vi "Interrogate_register.vi"(6 "Address override":i32, 8 "error in (no error)":errorcluster, 9 "UUT Index":i32, 10 "Register mutli-protocol location":T2={"General Parameter name"="", "MODBUS Register"=0, "Profibus"={"Friendly name"="", "PA"={"Slot"=0, "Index"=0}, "DP"={"Slot"=0, "Index"=0}, "Tag"=""}, "Fieldbus"={"Parameter name"="", "Fieldbus Block"="", "Fieldbus Tag"=""}, "data type"=enum."float", "DeviceNET"={"ClassId"=102, "InstanceId"=1, "AttributeId"=12}, "Cluster"={"address"=0, "Mode"=0}, "Length"=0} {"Cluster"."Mode" items=["None", "MODBUS", "HART", "Profibus DP", "Profibus PA", "Fieldbus", "DeviceNET"]}, 11 "HART in":refnum<class "HART.lvclass">) -> (0 "error out":errorcluster, 1 "Parameter name":string, 2 "output":sgl, 3 "HART out":refnum<class "HART.lvclass">, 4 "output cluster":T1)   [LabVIEW 2016, in "HART.lvclass"]
uses:
  HART.lvclass
  Typedef/comm_variable_definition.ctl
  Typedef/Comm_mode_and_address_type.ctl
  Typedef/Comm_mode_type_combo.ctl
  HART.lvclass/HART.ctl
  Protocol Class/Protocol.lvclass
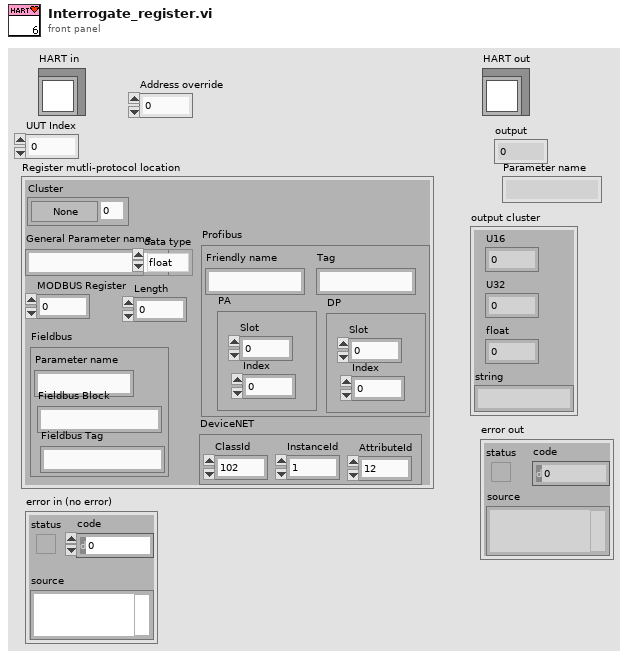
[diagram p1: front panel]
types:
  T1 = cluster{"U16":u16, "U32":u32, "float":sgl, "string":string}
  T2 = typedef "comm_variable_definition.ctl" = cluster{"General Parameter name":string, "MODBUS Register":i32, "Profibus":cluster{"Friendly name":string, "PA":cluster{"Slot":i32, "Index":i32}, "DP":cluster{"Slot":i32, "Index":i32}, "Tag":string}, "Fieldbus":cluster{"Parameter name":string, "Fieldbus Block":string, "Fieldbus Tag":string}, "data type":enum16{"float", "UINT", "UINT32", "STRING"}, "DeviceNET":cluster{"ClassId":u16, "InstanceId":u16, "AttributeId":u8}, "Cluster":T3, "Length":i32}
  T3 = typedef "Comm_mode_and_address_type.ctl" = cluster{"address":i32, "Mode":T4}
  T4 = typedef "Comm_mode_type_combo.ctl" = u16
  T5 = enum16{"None", "Coil", "Uint16", "Uint32", "Float"}
  T6 = enum16{"0-1-2-3", "2-3-0-1", "1-0-3-2", "3-2-1-0"}
  T7 = cluster{"Long address":u8[], "Short address":i32, "Switch index":i32}[]
  T8 = cluster{"Long address":u8[], "Short address":i32, "Switch index":i32}
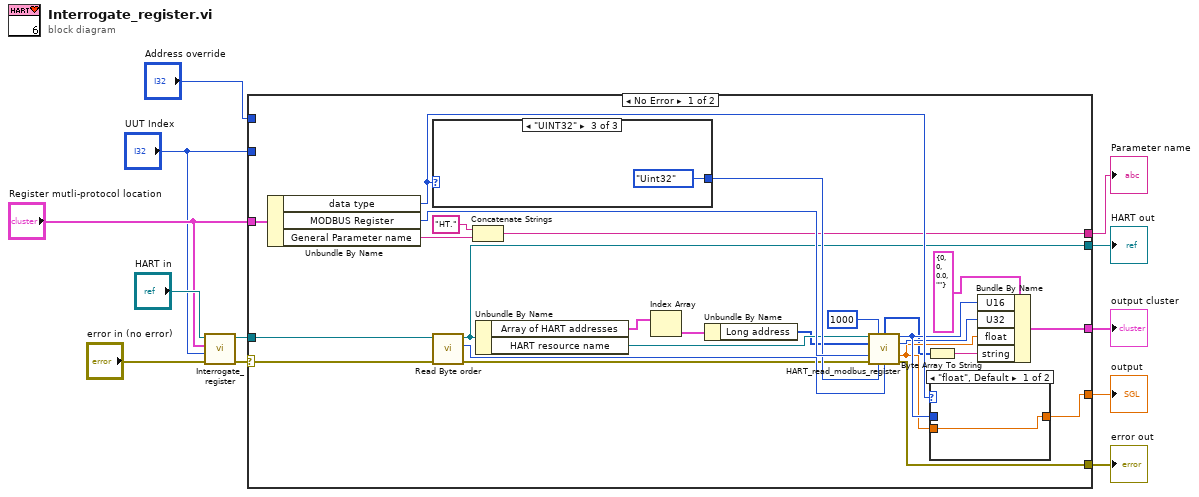
[diagram p0: block diagram]
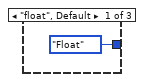
[diagram p3: hidden frame]
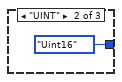
[diagram p4: hidden frame]
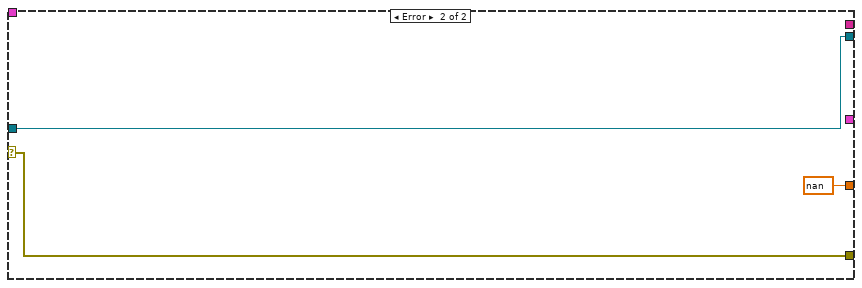
[diagram p5: hidden frame]
diagram:
  n1 = call-parent "Interrogate_register.vi"("error in (no error)"="error in (no error)", "UUT Index"="UUT Index", "Register mutli-protocol location"="Register mutli-protocol location", "Protocol in"="HART in") -> ("error out"=w10:errorcluster, "Protocol out"=w9:refnum<class "HART.lvclass">)  [unwired: 3 in, 3 out]
  n2 = case shown="No Error" w10 {
    selector: w10 -> [w14 w46]
    tunnel: "Register mutli-protocol location" -> [w38 _]
    tunnel: [w37 sgl nan ("type single")] -> w4
    tunnel: [w34 w46] -> w5
    tunnel: "UUT Index" -> [_ _]
    tunnel: w9 -> [w17 w44]
    tunnel: [w16 w44] -> w6
    tunnel: [w25 _] -> w3
    tunnel: "Address override" -> [_ _]
    tunnel: [w18 _] -> w1
    frame No Error {
      n3 = Unbundle By Name(w38) -> ("data type"=w36:enum16{"float", "UINT", "UINT32", "STRING"}, "MODBUS Register"=w35:i32, "General Parameter name"=w26:string)
      n4 = case shown="\"UINT32\"" w36 {
        tunnel: [T5."Float" ("data type") T5."Uint16" ("data type") T5."Uint32" ("data type")] -> w33
        frame "float", Default {
        }
        frame "UINT" {
        }
        frame "UINT32" {
        }
      }
      n5 = call-dynamic "Read Byte order.vi"("error in (no error)"=w14, "Protocol in"=w17) -> ("error out"=w13:errorcluster, "Byte order"=w15:T6, "Protocol out"=w16:refnum<class "HART.lvclass">)  [unwired: 7 in]
      n6 = Concatenate Strings("HT." ("Protocol name"), w26) -> (w25:string)
      n7 = Unbundle By Name(w16) -> ("Array of HART addresses"=w31:T7, "HART resource name"=w32:refnum<visa-resource-name>)
      n8 = Index Array(array=w31) -> (element=w30:T8)  [unwired: 1 in]
      n9 = Unbundle By Name(w30) -> ("Long address"=w29:u8[])
      n10 = call "HART_read_modbus_register.vi"("port number"=w32, "Max listen time\n(1000 ms)"=u32 1000 ("Max listen time\n(1000 ms)"), "address (array)"=w29, "MODBUS Reg."=w35, "error IN"=w13, "data type"=w33, "Byte order"=w15) -> ("Data bytes"=w20:u8[], "Unsigned 16 out"=w23:u16, "unsigned 32 out"=w22:u32, "floating point out"=w21:sgl, "error out"=w34:errorcluster)  [unwired: 1 in, 3 out]
      n11 = Byte Array To String(unsigned byte array=w20) -> (string=w19:string)
      n12 = case shown="\"float\", Default" w36 {
        tunnel: [w39 w40] -> w37
        tunnel: w21 -> [w39 _]
        tunnel: w23 -> [_ w40]
        frame "float", Default {
        }
        frame "UINT" {
        }
      }
      n13 = Bundle By Name(cluster=T1 {"U16"=0, "U32"=0, "float"=0.0, "string"=""} ("output cluster"), "U16"=w23, "U32"=w22, "float"=w21, "string"=w19) -> (w18:T1)
    }
    frame Error {
    }
  }
  "error out" <- w5
  "HART out" <- w6
  "output" <- w4
  "Parameter name" <- w3
  "output cluster" <- w1
